vi "main.vi"() -> ()   [LabVIEW 2020]
uses:
  <vilib>/picture/picture.llb/imagedata.ctl
  polar graph.ctl
  <vilib>/MakerHub/LINX/Public/Utilities/Open Serial.vi
  <vilib>/MakerHub/LINX/Public/Sensors/Motion/Servo/Servo Open One Channel.vi
  <vilib>/MakerHub/LINX/Public/Sensors/Motion/Servo/Servo Set Pulse Width One Channel.vi
  <vilib>/MakerHub/LINX/Public/Sensors/Motion/Servo/Servo Close One Channel.vi
  <vilib>/MakerHub/LINX/LMH-LINX.lvlib
  <vilib>/MakerHub/LINX/Public/Sensors/Motion/Servo/Servo.lvlib
  <vilib>/MakerHub/LINX/Public/Sensors/Distance/Ultrasonic/Ultrasonic.lvlib
  <vilib>/Analysis/NI_AALPro.lvlib
panel:
  out "In Range?":bool
  out "Distance":dbl
  in  "top left point(0, 0)":cluster{"x":i16, "y":i16}
  out "picture":picture
  out "Degrees":dbl
  in  "Servo":u8=6
  in  "Serial Port":refnum<visa-resource-name>="COM3"
  in  "Stop":bool
  # "Control"
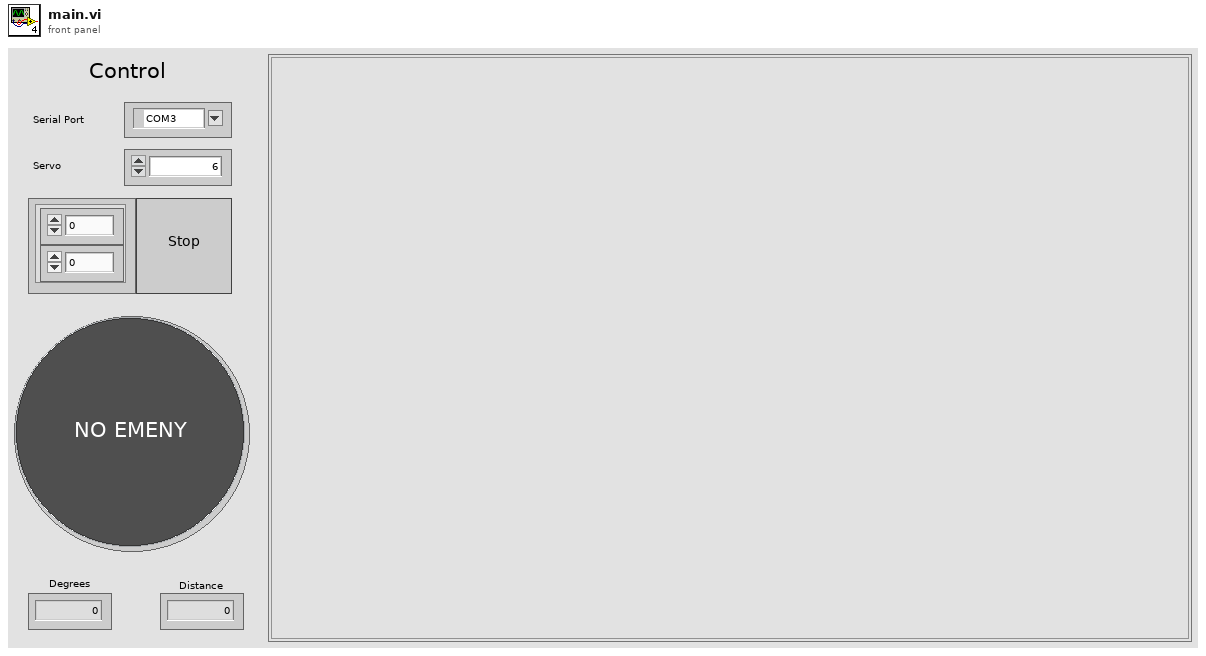
[diagram p1: front panel]
types:
  T1 = typedef "imagedata.ctl" = cluster{"image type":i32, "image depth":i32, "image":u8[], "mask":u8[], "colors":u32[], "Rectangle":cluster{"left":i16, "top":i16, "right":i16, "bottom":i16}}
  T2 = typedef "LMH-LINX.lvlib/LINX Ref.ctl" = cluster{"IO":T3, "Interface":T4, "LINX Device Config":T5}
  T3 = typedef "LMH-LINX.lvlib/Platform.ctl" = enum16{"Remote", "Local"}
  T4 = typedef "LMH-LINX.lvlib/Interface.ctl" = enum16{"Serial", "TCP"}
  T5 = typedef "LMH-LINX.lvlib/Device.lvlib/LINX Device Config.ctl" = cluster{"Interface":T4, "COM Port":refnum<visa-resource-name>, "TCP Configuration":T6, "Device Family":u8, "Device ID":u8, "Device Name":string, "TCP Ref":refnum<k5>, "Channels":T7}
  T6 = typedef "LMH-LINX.lvlib/Device.lvlib/TCP Config.ctl" = cluster{"IP Address":string, "Port":u16}
  T7 = typedef "LMH-LINX.lvlib/Channels.ctl" = cluster{"DI":u8[], "DO":u8[], "AI":u8[], "AO":u8[], "PWM":u8[], "QE":u8[], "UART":u8[], "I2C 2":u8[], "SPI":u8[], "CAN":u8[], "Servo":u8[], "AI Ref (V)":dbl, "AI Resolution (Bits)":u8, "AO Ref (V)":dbl, "AO Resolution (Bits)":u8}
  T8 = typedef "polar graph.ctl" = cluster{"maximum":dbl, "minimum":dbl, "clip to min":bool, "log?(F)":bool, "grid color":u32, "plot color":u32, "fmt and prec":cluster{"format":enum8{"Decimal", "Scientific", "Engineering", "Binary", "Octal", "Hex"}, "precision":u8}, "visible section":u16}
  T9 = typedef "LVBoundsTypeDef.ctl" = cluster{"Width":u32, "Height":u32}
  T10 = cluster{"pixel center":cluster{"x":i16, "y":i16}, "scale factors":cluster{"a":dbl, "b":dbl, "log?":bool}, "grid color":u32, "start angle":dbl, "end angle":dbl, "tick length":i16, "pixel radius":i32}
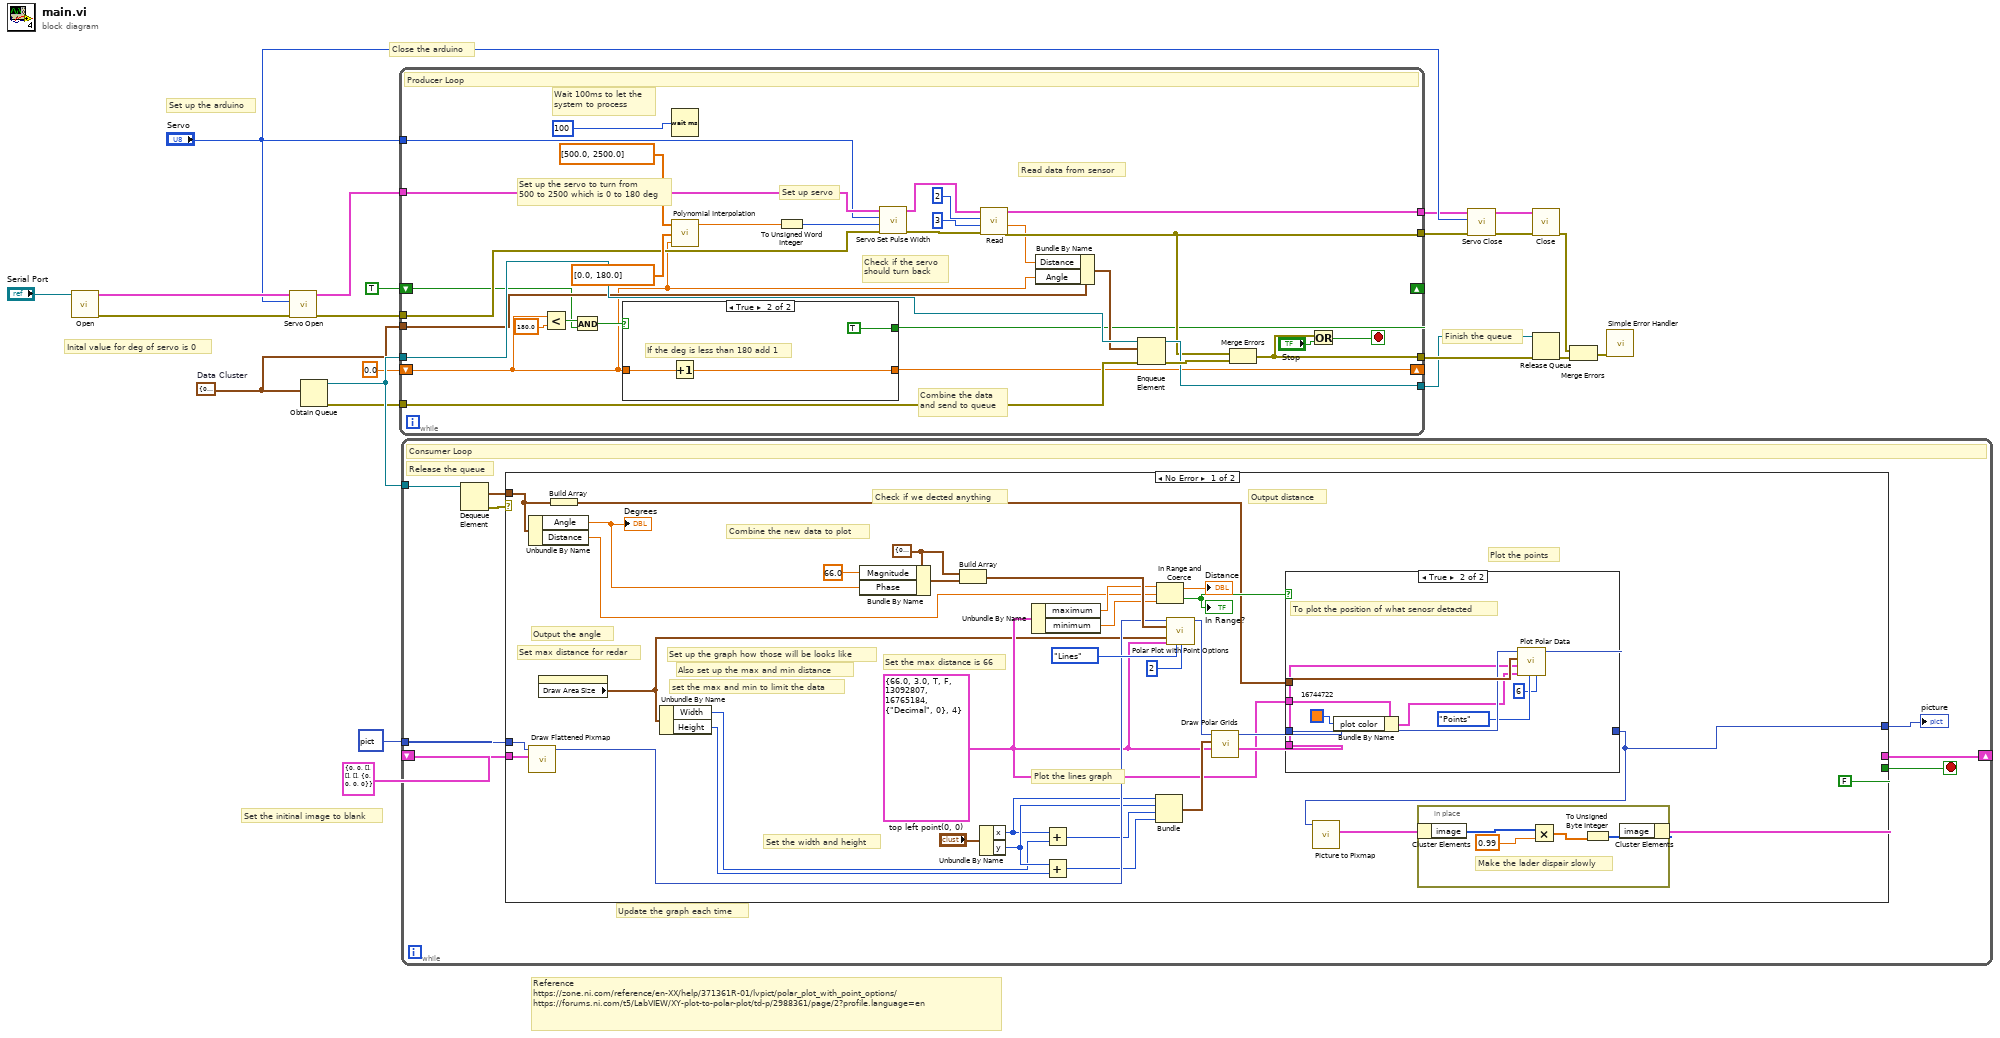
[diagram p0: block diagram]
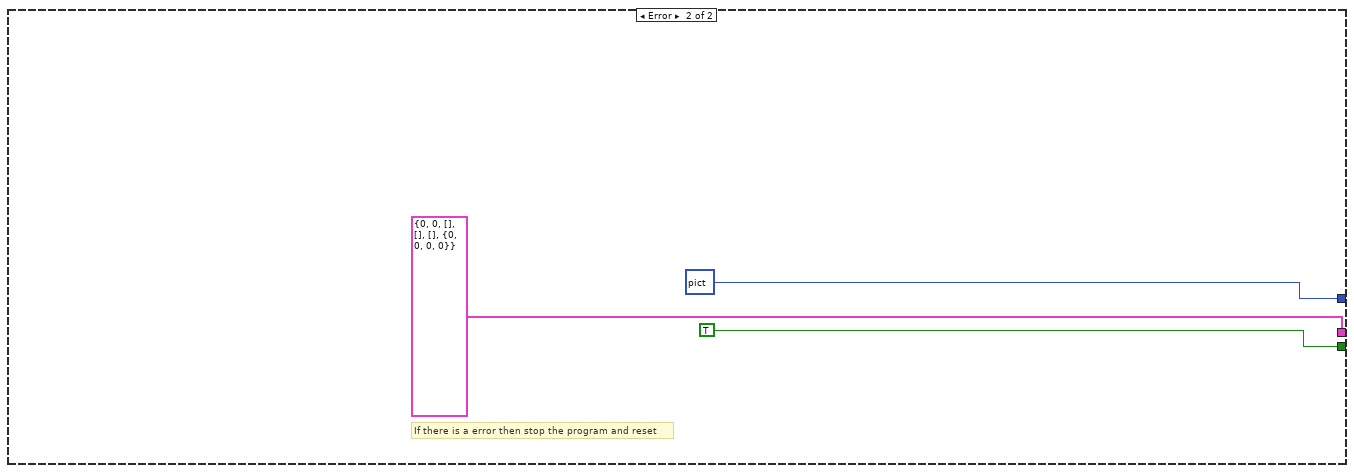
[diagram p3: hidden frame]
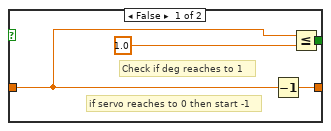
[diagram p4: hidden frame]
diagram:
  w8 = cluster{"Distance":dbl, "Angle":dbl} {"Distance"=0.0, "Angle"=0.0}  # Data Cluster
  # "Reference\nhttps://zone.ni.com/reference/en-XX/help/371361R-01/lvpict/polar_plot_with_point_options/\nhttps://forums.ni.com/t5/LabVIEW/XY-plot-to-polar-plot/td-p/2988361/page/2?profile.language=en"
  # "Set the initinal image to blank"
  # "Finish the queue"
  # "Close the arduino"
  # "Inital value for deg of servo is 0"
  # "Set up the arduino"
  n1 = call-poly <vilib>:"Open.vi"("Serial Port"="Serial Port") -> ("Error Out"=w18:errorcluster, "LINX Resource"=w19:T2)  [unwired: 8 in, 1 out]
  n2 = call-poly <vilib>:"Servo Open.vi"("Error In"=w18, "Servo Channel"="Servo", "LINX Resource"=w19) -> ("Error Out"=w16:errorcluster, "LINX Resource"=w17:T2)  [unwired: 7 in]
  n3 = Obtain Queue(element data type=w8) -> (queue out=w22:refnum<queue>, error out=w21:errorcluster)  [unwired: 4 in, 1 out]
  n4 = while {
    tunnel: w22 -> [w53]
    tunnel: w21 -> [w52]
    tunnel: "Servo" -> [w32]
    tunnel: w17 -> [w33]
    tunnel: w16 -> [w34]
    tunnel: [w48] -> w12
    tunnel: [w47] -> w11
    tunnel: [w43] -> w10
    tunnel: [w42] -> w9
    tunnel: w8 -> [w40]
    shift-right: [w24] -> _
    shift-left: 0.0 -> [w23]
    shift-right: [w28] -> _
    shift-left: TRUE -> [w26]
    stop <- w49 stop-if-true
    # "Wait 100ms to let the \nsystem to process"
    # "Combine the data \nand send to queue"
    # "Read data from sensor"
    # "Set up servo"
    # "Check if the servo\nshould turn back"
    # "Set up the servo to turn from \n500 to 2500 which is 0 to 180 deg"
    # "Producer Loop"
    n5 = Less?(x=w23, y=180.0) -> (x < y?=w27:bool)
    n6 = And(x=w27, y=w26) -> (x .and. y?=w25:bool)
    n7 = case shown="True" w25 {
      tunnel: w23 -> [w56 w60]
      tunnel: [w57 w59] -> w24
      tunnel: [w54 TRUE] -> w28
      frame False {
        # "Check if deg reaches to 1"
        # "if servo reaches to 0 then start -1"
        n8 = Decrement(x=w56) -> (x-1=w57:dbl)
        n9 = Less Or Equal?(x=w56, y=1.0) -> (x <= y?=w54:bool)
      }
      frame True {
        # "If the deg is less than 180 add 1"
        n10 = Increment(x=w60) -> (x+1=w59:dbl)
      }
    }
    n11 = Wait (ms)(milliseconds to wait=u32 100) -> ()  [unwired: 1 out]
    n12 = call <vilib>:"Polynomial Interpolation.vi"("x value"=w23, "X"=dbl[] [0.0, 180.0], "Y"=dbl[] [500.0, 2500.0]) -> ("interpolation value"=w38:dbl)  [unwired: 2 out]
    n13 = To Unsigned Word Integer(number=w38) -> (unsigned 16bit integer=w35:u16)
    n14 = call-poly <vilib>:"Servo Set Pulse Width.vi"("Error In"=w34, "Pulse Width (uS)"=w35, "Servo Channel"=w32, "LINX Resource"=w33) -> ("Error Out"=w30:errorcluster, "LINX Resource"=w31:T2)  [unwired: 6 in]
    n15 = call <vilib>:"Read.vi"("Error In"=w30, "DO Channel"=u8 3, "DI Channel"=u8 2, "LINX Resource"=w31) -> ("Error Out"=w42:errorcluster, "Centimeters"=w41:dbl, "LINX Resource"=w43:T2)  [unwired: 4 in, 1 out]
    n16 = Bundle By Name(cluster=w40, "Distance"=w41, "Angle"=w23) -> (w39:cluster{"Distance":dbl, "Angle":dbl})
    n17 = Enqueue Element(queue=w53, element=w39, error in (no error)=w52) -> (queue out=w47:refnum<queue>, error out=w51:errorcluster)  [unwired: 1 in, 1 out]
    n18 = Merge Errors(w42, w51) -> (w48:errorcluster)
    n19 = Or(x=w48, y="Stop") -> (x .or. y?=w49:bool)
  }
  n20 = while {
    tunnel: w22 -> [w66]
    tunnel: picture data[5B] ("picture") -> [w64]
    shift-right: [w61] -> _
    shift-left: T1 {"image type"=0, "image depth"=0, "image"=[], "mask"=[], "colors"=[], "Rectangle"={"left"=0, "top"=0, "right"=0, "bottom"=0}} ("image data") -> [w63]
    stop <- w67 stop-if-true
    # "Update the graph each time"
    # "Release the queue"
    # "Consumer Loop"
    n21 = Dequeue Element(queue=w66) -> (element=w65:cluster{"Distance":dbl, "Angle":dbl}, error out=w68:errorcluster)  [unwired: 2 in, 2 out]
    n22 = case shown="No Error" w68 {
      tunnel: [FALSE TRUE] -> w67
      tunnel: w65 -> [w75 _]
      tunnel: w64 -> [w93 _]
      tunnel: w63 -> [w92 _]
      tunnel: [w72 picture data[5B] ("new picture")] -> w62
      tunnel: [w70 T1 {"image type"=0, "image depth"=0, "image"=[], "mask"=[], "colors"=[], "Rectangle"={"left"=0, "top"=0, "right"=0, "bottom"=0}} ("image data")] -> w61
      frame No Error {
        w96 = cluster{"Magnitude":dbl, "Phase":dbl} {"Magnitude"=0.0, "Phase"=0.0} ("Line")
        w73 = T8 {"maximum"=66.0, "minimum"=3.0, "clip to min"=TRUE, "log?(F)"=FALSE, "grid color"=13092807, "plot color"=16765184, "fmt and prec"={"format"=enum."Decimal", "precision"=0}, "visible section"=4} ("polar attributes")
        # "Plot the lines graph"
        # "Plot the points"
        # "Output distance"
        # "Also set up the max and min distance"
        # "set the max and min to limit the data"
        # "Set the width and height"
        # "Set the max distance is 66"
        # "Combine the new data to plot"
        # "Output the angle"
        # "Set max distance for redar"
        # "Check if we dected anything"
        # "Set up the graph how those will be looks like"
        n23 = Unbundle By Name(w75) -> ("Angle"=w99:dbl, "Distance"=w80:dbl)
        "Degrees" <- w99
        n24 = call <vilib>:"Draw Flattened Pixmap.vi"("image data"=w92, "picture"=w93) -> ("new picture"=w91:picture)  [unwired: 7 in]
        n25 = property on="picture" class="Pict"() -> ("Draw Area Size"=w69:T9)  [unwired: 2 in, 2 out]
        n26 = Build Array(w75) -> (w74:cluster{"Distance":dbl, "Angle":dbl}[])
        n27 = Unbundle By Name(w69) -> ("Width"=w85:u32, "Height"=w86:u32)
        n28 = Bundle By Name(cluster=w96, "Magnitude"=66.0, "Phase"=w99) -> (w97:cluster{"Magnitude":dbl, "Phase":dbl})
        n29 = Build Array(w96, w97) -> (w95:cluster{"Magnitude":dbl, "Phase":dbl}[])
        n30 = Unbundle By Name("top left point(0, 0)") -> ("x"=w87:i16, "y"=w88:i16)
        n31 = Unbundle By Name(w73) -> ("maximum"=w82:dbl, "minimum"=w81:dbl)
        n32 = Add(x=w87, y=w85) -> (x+y=w89:u32)
        n33 = Add(x=w88, y=w86) -> (x+y=w90:u32)
        n34 = Bundle("x"=w87, "y"=w88, w89, w90) -> (w83:cluster{"x":i16, "y":i16, u32, u32})  [unwired: 1 in]
        n35 = In Range and Coerce(upper limit=w82, x=w80, lower limit=w81) -> (coerced(x)=→"Distance":dbl, In Range?=w78:bool)
        "In Range?" <- w78
        n36 = call <vilib>:"Polar Plot with Point Options.vi"("picture"=w91, "data array [mag, phase (deg)]"=w95, "dimensions (w,h)"=w69, "polar attributes"=w73, "Lines/Points"=enum16{"Lines", "Points"}."Lines", "Size"=u16 2) -> ("new picture"=w94:picture)  [unwired: 9 in]
        n37 = call <vilib>:"Draw Polar Grids.vi"("polar attributes"=w73, "rect"=w83, "picture"=w94) -> ("grid measurements"=w76:T10, "new picture"=w77:picture)  [unwired: 7 in]
        n38 = case shown="True" w78 {
          tunnel: w77 -> [w107 w115]
          tunnel: w76 -> [_ w114]
          tunnel: w74 -> [_ w116]
          tunnel: w73 -> [_ w113]
          tunnel: [w107 w110] -> w72
          frame False {
          }
          frame True {
            # "To plot the position of what senosr detacted"
            n39 = Bundle By Name(cluster=w113, "plot color"=u32 16744722) -> (w111:T8)
            n40 = call <vilib>:"Plot Polar Data.vi"("Size"=u16 6, "Lines/Points"=enum16{"Lines", "Points"}."Points", "polar attributes"=w111, "grid measurements"=w114, "polar data"=w116, "picture"=w115) -> ("new picture"=w110:picture)  [unwired: 3 in]
          }
        }
        n41 = call <vilib>:"Picture to Pixmap.vi"("picture"=w72) -> ("image data"=w71:T1)  [unwired: 9 in, 1 out]
        n42 = in-place {
          # "Make the lader dispair slowly"
          n43 = in-place-cluster #1(w71) -> ("image"=w105:u8[])
          n44 = Multiply(x=w105, y=0.99) -> (x*y=w104:dbl[])
          n45 = To Unsigned Byte Integer(number=w104) -> (unsigned 8bit integer=w103:u8[])
          n46 = in-place-cluster #1("image"=w103) -> (w70:T1)
        }
      }
      frame Error {
        # "If there is a error then stop the program and reset"
      }
    }
    "picture" <- w62
  }
  n47 = call-poly <vilib>:"Servo Close.vi"("Error In"=w9, "Servo Channel"="Servo", "LINX Resource"=w10) -> ("Error Out"=w15:errorcluster, "LINX Resource"=w14:T2)  [unwired: 7 in]
  n48 = call <vilib>:"Close.vi"("Error In"=w15, "LINX Resource"=w14) -> ("Error Out"=w7:errorcluster)  [unwired: 9 in]
  n49 = Release Queue(queue=w11, error in (no error)=w12) -> (error out=w6:errorcluster)  [unwired: 1 in, 2 out]
  n50 = Merge Errors(w7, w6) -> (w5:errorcluster)
  n51 = call <vilib>:"Simple Error Handler.vi"("error in (no error)"=w5) -> ()  [unwired: 4 in, 5 out]
